vi "Shooter Calibrations.vi"() -> ()   [LabVIEW 2016]
panel:
  out "Long Range Shooter Wheel Speed (rpm)":dbl
  in  "Shooter Calibrations File Location":path=path "C:/ni-rt/startup/ShooterCalibrations.txt"
  out "Time Duration Within Shooter Wheel Speed Acceptable Error (ms)":dbl
  out "Shooter Wheel Speed Acceptable Error (rpm)":dbl
  out "Close Range Shooter Wheel Speed (rpm)":dbl
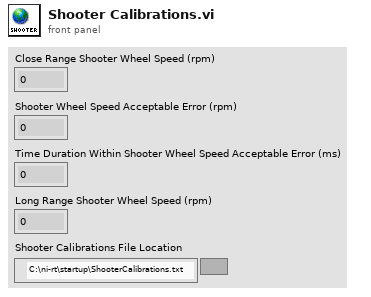
[diagram p1: front panel]
diagram:
